vi "Apply OCP Limit.vi"(8 "error in":errorcluster, 11 "6032A in":refnum<class "6032A.lvclass">) -> (0 "error out":errorcluster, 3 "6032A out":refnum<class "6032A.lvclass">)   [LabVIEW 2019, in "6032A.lvlib" / "6032A.lvclass"]
uses:
  Library/6032A.lvclass
  C:/Users/Public/Documents/Development/builds/Instruments/PowerSupply.lvlibp/Library/PowerSupply.lvclass
  Library/6032A.lvclass/6032A.ctl
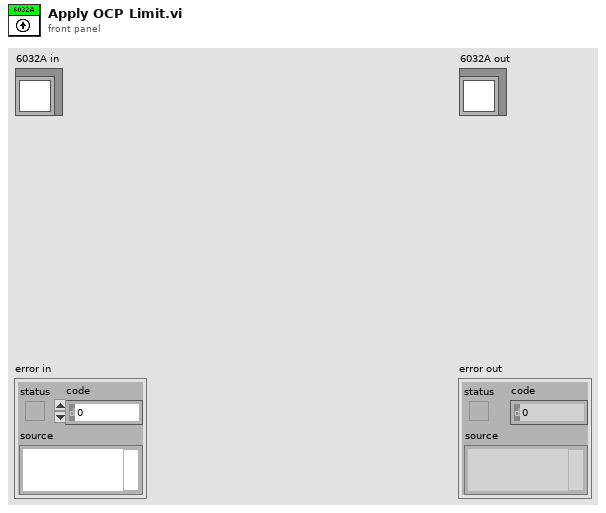
[diagram p1: front panel]
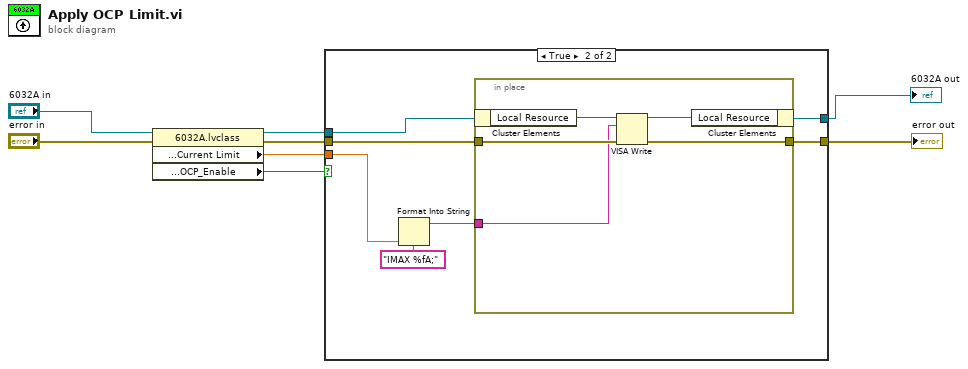
[diagram p0: block diagram]
diagram:
  n1 = property class="6032A.lvclass"(reference="6032A in", error in="error in") -> (reference out=w4:refnum<class "6032A.lvclass">, error out=w3:errorcluster, "Accessors:Setting:Protection:Current Limit"=w6:dbl, "Accessors:Setting:Protection:OCP_Enable"=w5:bool)
  n2 = case shown="True" w5 {
    tunnel: w6 -> [_ w16]
    tunnel: w4 -> [w10 w15]
    tunnel: w3 -> [w9 w14]
    tunnel: [w10 w13] -> w1
    tunnel: [w9 w12] -> w2
    frame False {
    }
    frame True {
      n3 = Format Into String(format string="IMAX %fA;", w16) -> (resulting string=w11:string)  [unwired: 2 in, 1 out]
      n4 = in-place {
        in-place-border: w14 -> [w21]
        in-place-border: [w19] -> w12
        in-place-border: w11 -> [w18]
        n5 = in-place-cluster #1(w15) -> ("Local Resource"=w22:refnum<visa-resource-name>)
        n6 = VISA Write(VISA resource name=w22, write buffer=w18, error in (no error)=w21) -> (VISA resource name out=w20:refnum<visa-resource-name>, error out=w19:errorcluster)  [unwired: 1 out]
        n7 = in-place-cluster #1("Local Resource"=w20) -> (w13:refnum<class "6032A.lvclass">)
      }
    }
  }
  "error out" <- w2
  "6032A out" <- w1
